vi "Set Re-entrancy for VIs in a Folder.vi"(6 "Exclude Pattern":string="LV2", 8 "error in (no error)":errorcluster, 9 "Reentrancy Type":T1(ring), 10 "Is Reentrant?":bool, 11 "VI Folder":path) -> (0 "error out":errorcluster, 2 "VIs with Errors":path[](array[path]), 3 "VI List":path[](array[path]))   [LabVIEW 2016, in "SLL Scripting.lvlib"]
doc: "This VI can be used to find the list of broken VIs in a folder. This also returns VIs which are of higher LabVIEW version than the currently used LabVIEW version."
uses:
  SLL Scripting.lvlib
  <vilib>/regexp/Match Regular Expression.xnode
panel:
  out "Progress":i32
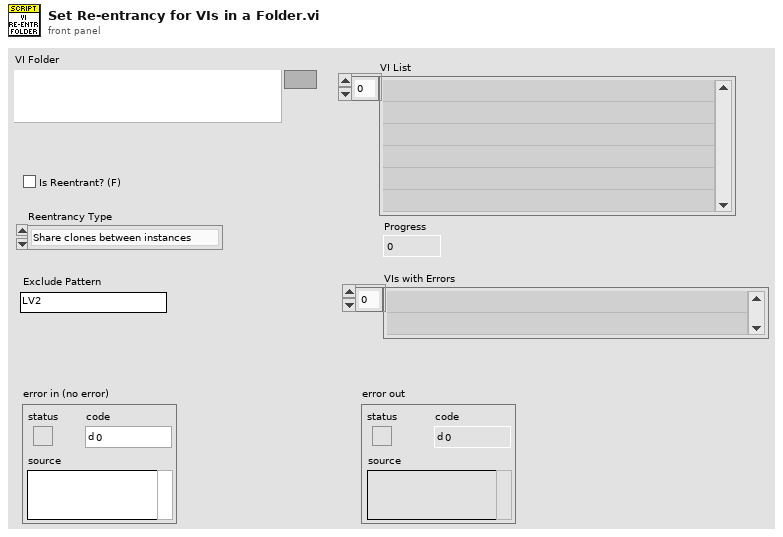
[diagram p1: front panel]
types:
  T1 = enum16{"Share clones between instances", "Preallocate clone for each instance"}
  T2 = enum32{"invalid VI type", "Standard VI", "Control VI", "Global VI", "Polymorphic VI", "Configuration VI", "SubSystem", "Facade VI", "Method VI", "Statechart Diagram VI"}
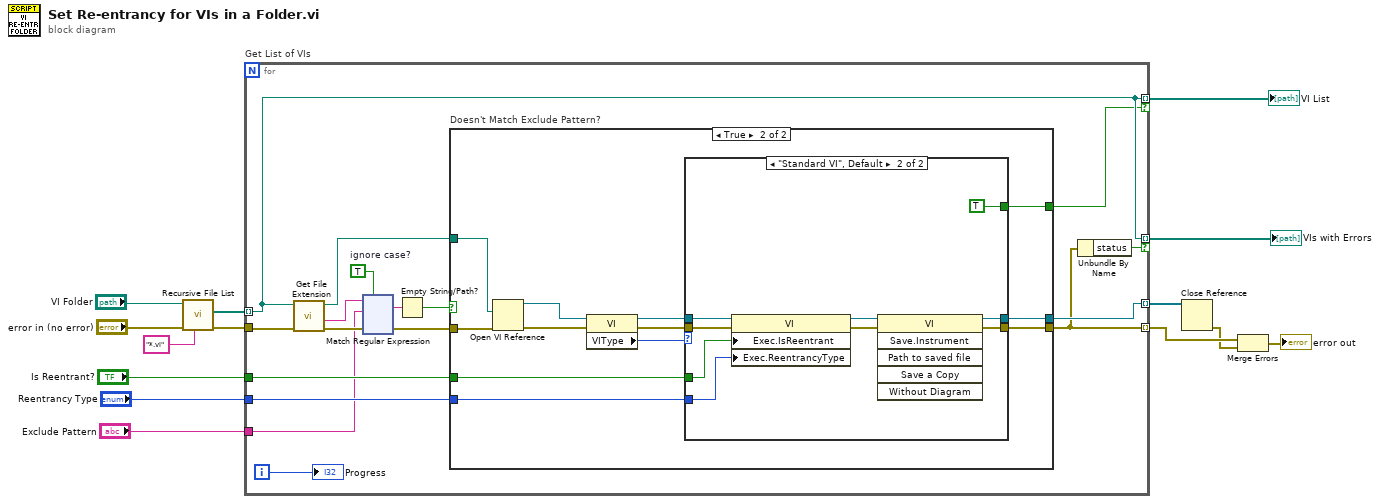
[diagram p0: block diagram]
diagram:
  n1 = call <vilib>:"Recursive File List.vi"("pattern"="*.vi", "error in (no error)"="error in (no error)", "Folder Path"="VI Folder") -> ("error out"=w8:errorcluster, "All Files in Dir"=w11:path[])  [unwired: 4 in, 3 out]
  n2 = for "Get List of VIs" {
    tunnel: [w30] -> w14 mode=indexing
    tunnel: w11 -> [w24] mode=indexing
    tunnel: [w24] -> w10 mode=indexing if=w15
    tunnel: w8 -> [w25]
    tunnel: [w27] -> w7 mode=indexing
    tunnel: "Reentrancy Type" -> [w29]
    tunnel: "Is Reentrant?" -> [w28]
    tunnel: [w24] -> w2 mode=indexing if=w26
    tunnel: "Exclude Pattern" -> [w18]
    i -> [w31]
    w20 = TRUE  # ignore case?
    n3 = call <vilib>:"Get File Extension.vi"("error in (no error)"=w25, "file"=w24) -> ("error out"=w22:errorcluster, "filename without extension"=w19:string, "dup file"=w23:path)  [unwired: 5 in, 2 out]
    n4 = xnode "Match Regular Expression"("input string"=w19, "regular expression"=w18, "error in"=w22, "ignore case? (F)"=w20) -> ("whole match"=w17:string, "error out"=w21:errorcluster)  [unwired: 2 in, 3 out]
    n5 = Empty String/Path?(string/path=w17) -> (empty?=w16:bool)
    n6 = case "Doesn't Match Exclude Pattern?" shown="True" w16 {
      tunnel: [_ w158] -> w30
      tunnel: w29 -> [_ w157]
      tunnel: w28 -> [_ w156]
      tunnel: [w146 w155] -> w27
      tunnel: w23 -> [_ w154]
      tunnel: w21 -> [w146 w153]
      tunnel: [_ w147] -> w15
      frame False {
      }
      frame True {
        n7 = Open VI Reference(vi path=w154, error in (no error)=w153) -> (vi reference=w151:refnum<vi>, error out=w152:errorcluster)  [unwired: 4 in]
        n8 = property class="VI"(reference=w151, error in=w152) -> (reference out=w150:refnum<vi>, error out=w149:errorcluster, "VIType"=w148:T2)
        n9 = case shown="\"Standard VI\", Default" w148 {
          tunnel: [w159 w167] -> w158
          tunnel: w157 -> [_ w166]
          tunnel: w156 -> [_ w165]
          tunnel: [w160 w164] -> w155
          tunnel: w150 -> [w159 w163]
          tunnel: w149 -> [w160 w162]
          tunnel: [_ TRUE] -> w147
          frame "Polymorphic VI" {
            # "Note: Polymorphic VIs will result in error when setting the re-entrancy setting"
            # "Ignoring for Polymorphic VIs"
          }
          frame "Standard VI", Default {
            n10 = property class="VI"(reference=w163, error in=w162, "Exec.IsReentrant"=w165, "Exec.ReentrancyType"=w166) -> (reference out=w168:refnum<vi>, error out=w169:errorcluster)
            n11 = invoke class="VI" method="Save.Instrument"(reference=w168, error in=w169) -> (reference out=w167:refnum<vi>, error out=w164:errorcluster)  [unwired: 4 in, 4 out]
          }
        }
      }
    }
    n12 = Unbundle By Name(w27) -> ("status"=w26:bool)
    "Progress" <- w31
  }
  "VI List" <- w10
  "VIs with Errors" <- w2
  n13 = Close Reference(reference=w14) -> (error out=w6:errorcluster)  [unwired: 1 in]
  n14 = Merge Errors(w7, w6) -> (→"error out":errorcluster)
